vi "4155C Write array to file.vi"(0 "Byte Stream File Refnum":refnum<file>, 1 "Header":string[](array[string]), 2 "Data Array":ext[][](array[numeric]) format="%.6e", 3 "error in (no error)":errorcluster, 4 "Separator":string="\t") -> (5 "dup refnum":refnum<file>, 6 "error out":errorcluster)   [LabVIEW 2016]
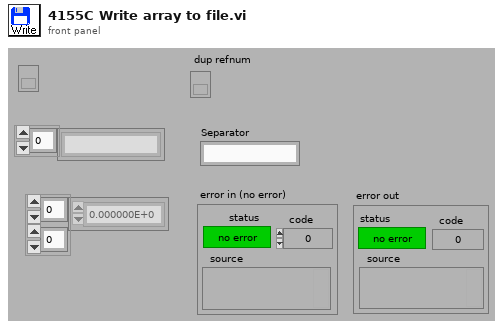
[diagram p1: front panel]
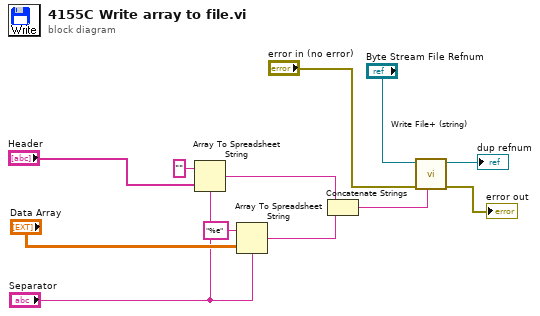
[diagram p0: block diagram]
diagram:
  n1 = Array To Spreadsheet String(delimiter (Tab)="Separator", array="Header", 3:"" ("format string")) -> (spreadsheet string=w8:string)
  n2 = Array To Spreadsheet String(delimiter (Tab)="Separator", array="Data Array", 3:"%e" ("format string")) -> (spreadsheet string=w9:string)
  n3 = Concatenate Strings(w8, w9) -> (w5:string)
  n4 = call <vilib>:"Write File+ (string).vi"("string"=w5, "error in (no error)"="error in (no error)", "refnum"="Byte Stream File Refnum") -> ("error out"=→"error out":errorcluster, "dup refnum"=→"dup refnum":refnum<file>)  [unwired: 4 in, 1 out]
